vi "Autonomous Independent.vi"() -> ()   [LabVIEW 2018]
doc: "This VI is called when autonomous begins, and will automatically be terminated when autonomous ends. You can carry out timed or sensor driven robot movement independently without needing to return to the caller."
uses:
  <vilib>/Rock Robotics/WPI/Solenoid/WPI_SolenoidValue.ctl
  <vilib>/Rock Robotics/WPI/Utilities/WPI_GetSetVariantRefNum.vi
  <vilib>/Rock Robotics/WPI/Solenoid/WPI_SolenoidSetEnum.vi
  <vilib>/Rock Robotics/Network Tables/NT Write Number.vi
  <vilib>/Rock Robotics/Network Tables/NT Write Boolean Array.vi
  <vilib>/Rock Robotics/Network Tables/NT Write Numeric Array.vi
  <vilib>/Rock Robotics/WPI/RobotDrive/WPI_RobotDriveArcadeDrive_Standard(NoSaturation).vi
  <vilib>/Rock Robotics/Network Tables/NT Read String.vi
panel:
  out "Current Movement, for debugging":T1 {"Y Joystick Value" scale=1.0..-1.0; "X Joystick Value" scale=-1.0..1.0}
  in  "Array of robot movements by from the robot":T2(array[cluster])=[{"X Joystick Value"=0.39393939393939403, "Y Joystick Value"=0.0, "Delay (sec)"=1.0, "Movement Name"="turn"}, {"X Joystick Value"=-0.3737373737373737, "Y Joystick Value"=0.0, "Delay (sec)"=1.0, "Movement Name"="turn back"}] {"Y Joystick Value" scale=1.0..-1.0; "X Joystick Value" scale=-1.0..1.0}
  # "Be sure to right-click and choose Data Operations>>Make Current Value default if you want to save the array values with the VI"
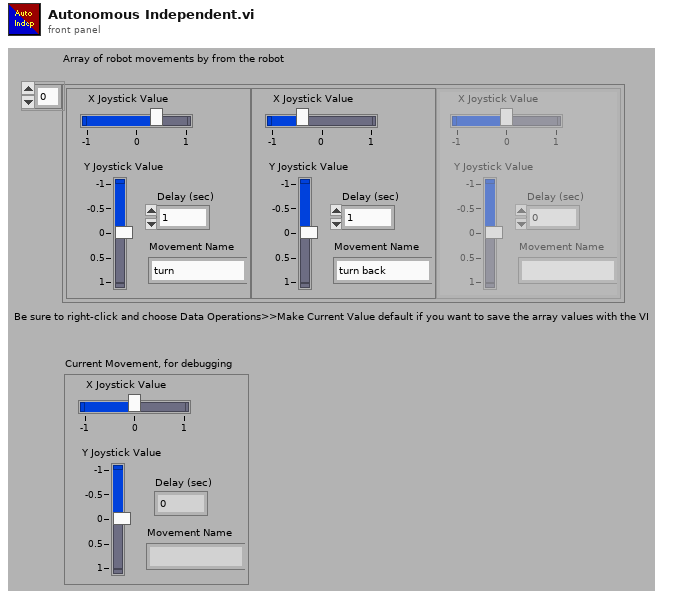
[diagram p1: front panel]
types:
  T1 = cluster{"X Joystick Value":dbl, "Y Joystick Value":dbl, "Delay (sec)":dbl, "Movement Name":string}
  T2 = cluster{"X Joystick Value":dbl, "Y Joystick Value":dbl, "Delay (sec)":dbl, "Movement Name":string}[]
  T3 = typedef "WPI_SolenoidValue.ctl" = enum16{"Off", "On", "Forward", "Reverse"}
  T4 = typedef "WPI_JoystickDevRef.ctl" = cluster{"Device":T5}
  T5 = typedef "WPI_JoystickDeviceEnum.ctl" = enum16{"USB 0", "USB 1", "USB 2", "USB 3", "USB 4", "USB 5"}
  T6 = typedef "WPI_SolenoidDevRef.ctl" = cluster{"DevStatus":errorcluster, "Pneumatics Control Module":u8, "Forward Solenoid Channel":T7, "Reverse Solenoid Channel":T7}
  T7 = typedef "WPI_SolenoidChannel.ctl" = enum8{"Solenoid 0", "Solenoid 1", "Solenoid 2", "Solenoid 3", "Solenoid 4", "Solenoid 5", "Solenoid 6", "Solenoid 7", "Invalid"}
  T8 = typedef "WPI_RobotDriveDevRef.ctl" = cluster{"DevStatus":errorcluster, "Motors[]":T9[], "Square Inputs":bool, "Max Output":dbl}
  T9 = typedef "WPI_MotorControlDeviceRef.ctl" = cluster{"DeviceStatus":errorcluster, "Type":T10, "PWM":cluster{"PWM Channel":T11, "DeadBand":T12}, "CAN":cluster{"Device Number":u8, "SetOutput VI Ref":variant, "GetOutput VI Ref":variant, "Enable VI Ref":variant, "Disable VI Ref":variant, "Data":variant}, "Invert":bool, "DIO PWM":cluster{"PWM \"Enable\" Channel":T11, "DIOChannel":T13, "PWM Rate":dbl}}
  T10 = typedef "WPI_MotorControlType.ctl" = enum16{"PWM", "CAN", "DIO PWM"}
  T11 = typedef "FPGA_DIOPWMChannel.ctl" = enum8{"PWM 0", "PWM 1", "PWM 2", "PWM 3", "PWM 4", "PWM 5", "PWM 6", "PWM 7", "PWM 8", "PWM 9", "PWM MXP 0", "PWM MXP 1", "PWM MXP 2", "PWM MXP 3", "PWM MXP 4", "PWM MXP 5", "PWM MXP 6", "PWM MXP 7", "PWM MXP 8", "PWM MXP 9", "Invalid"}
  T12 = typedef "WPI_PWMDeadband.ctl" = cluster{"Name":string, "maxPositivePwm":i32, "minPositivePwm":i32, "centerPwm":i32, "maxNegativePwm":i32, "minNegativePwm":i32, "angularRange":u16}
  T13 = typedef "FPGA_DIOChannel.ctl" = enum8{"DIO 0", "DIO 1", "DIO 2", "DIO 3", "DIO 4", "DIO 5", "DIO 6", "DIO 7", "DIO 8", "DIO 9", "DIO MXP 0", "DIO MXP 1", "DIO MXP 2", "DIO MXP 3", "DIO MXP 4", "DIO MXP 5", "DIO MXP 6", "DIO MXP 7", "DIO MXP 8", "DIO MXP 9", "DIO MXP 10", "DIO MXP 11", "DIO MXP 12", "DIO MXP 13", "DIO MXP 14", "DIO MXP 15", "SPI Port CS1", "SPI Port CS2", "SPI Port CS3", "SPI Port MISO", "SPI Port MOSI", "Invalid"}
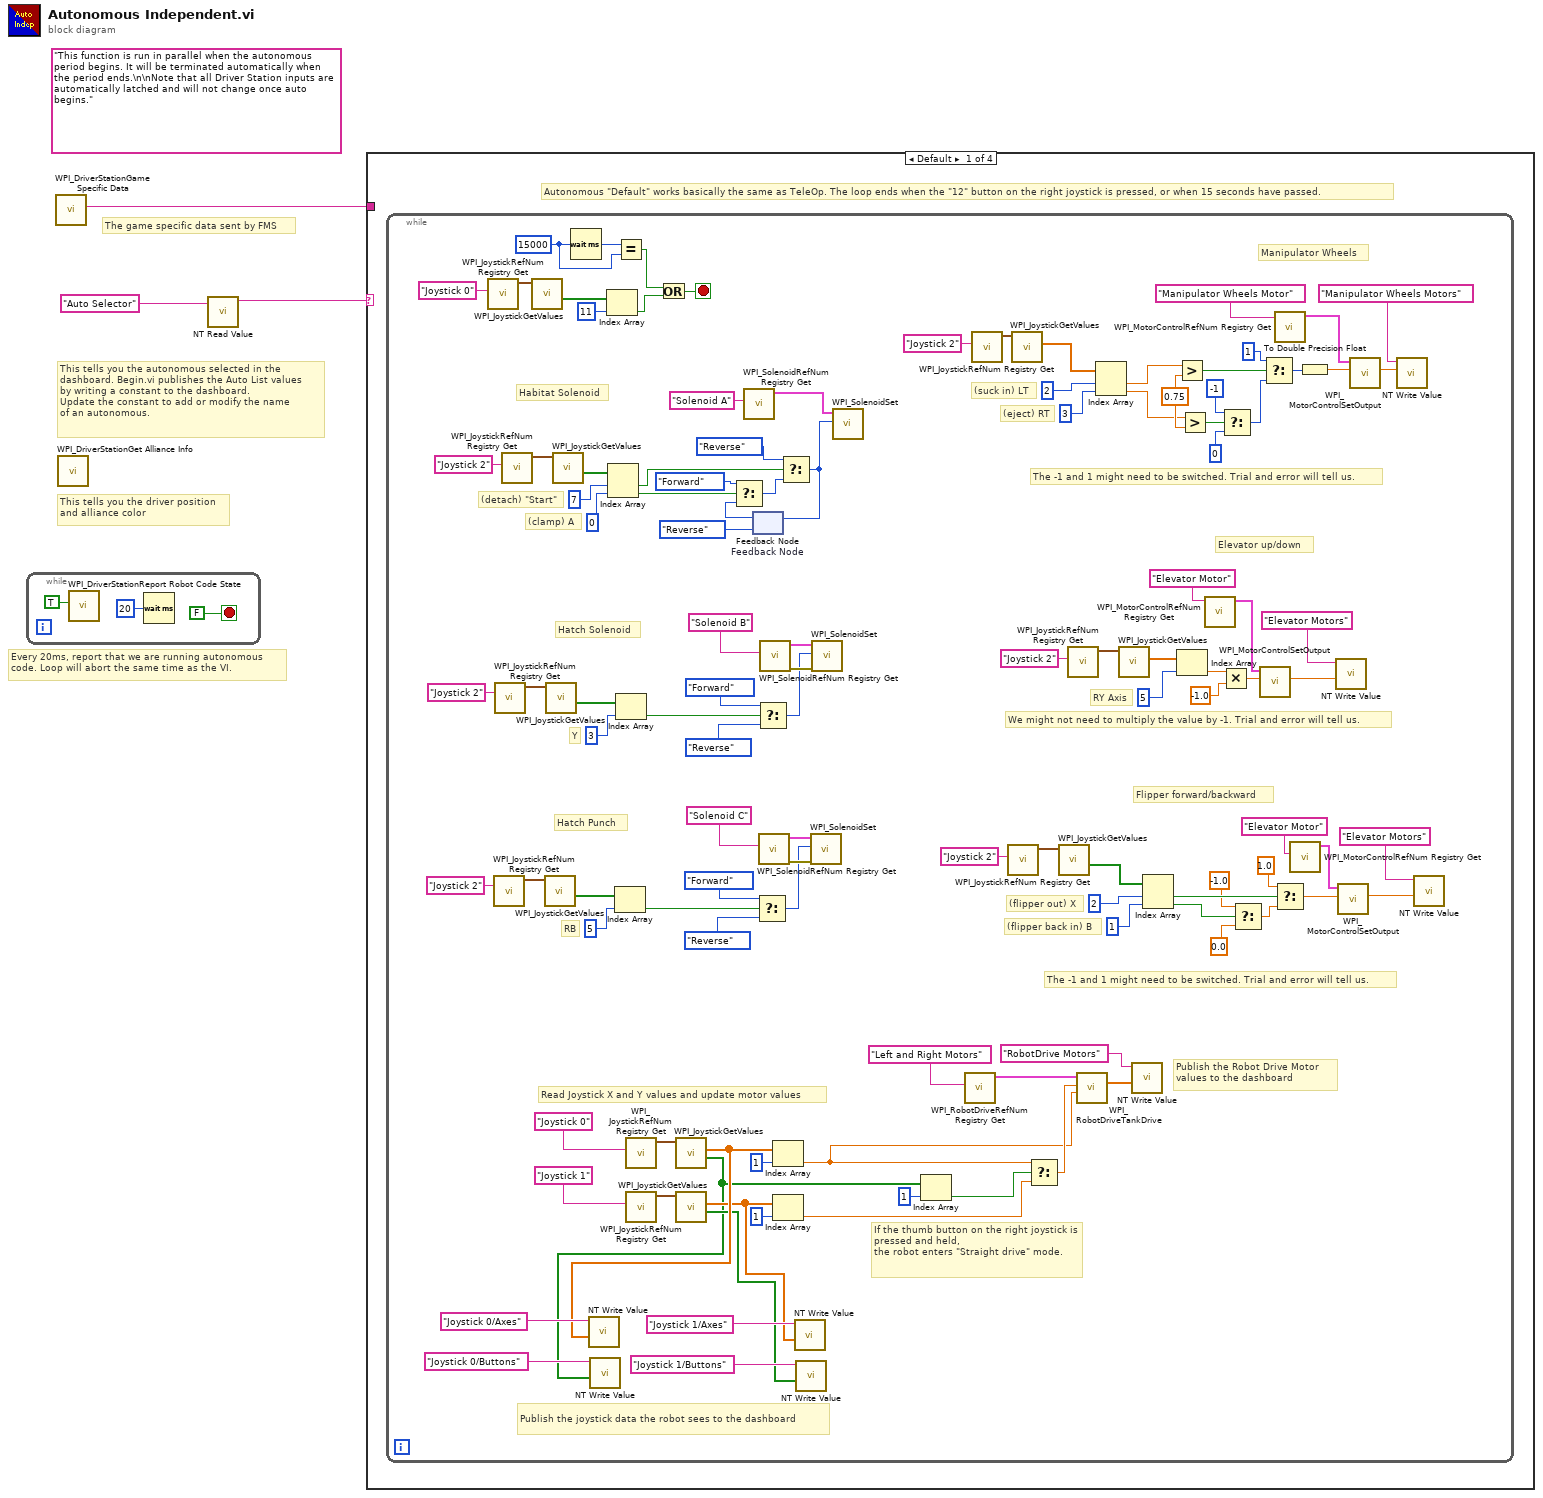
[diagram p0: block diagram]
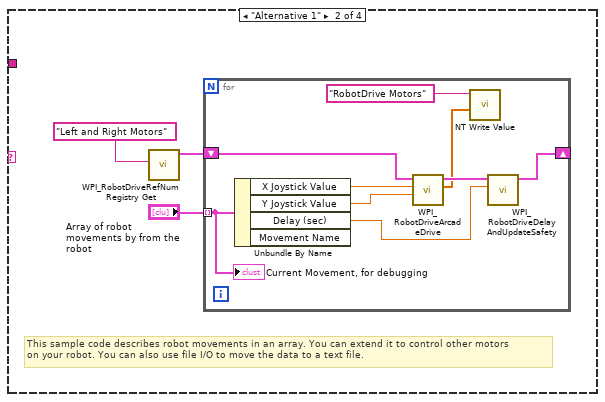
[diagram p2: hidden frame]
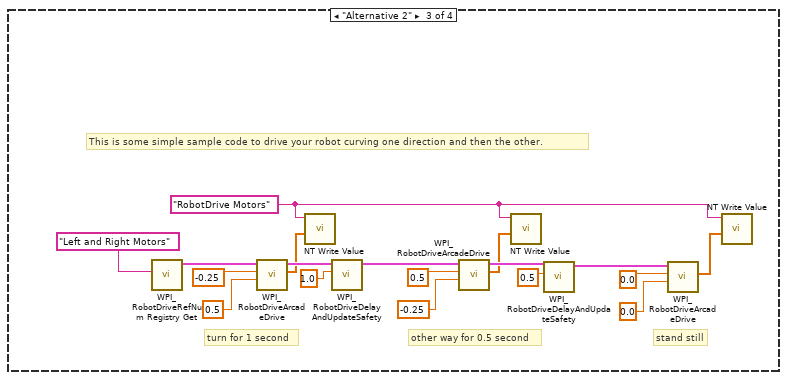
[diagram p3: hidden frame]
diagram:
  (unwired) "This function is run in parallel when the autonomous period begins. It will be terminated automatically when the period ends.\n\nNote that all Driver Station inputs are automatically latched and will not change once auto begins."
  # "The game specific data sent by FMS"
  # "This tells you the autonomous selected in the \ndashboard. Begin.vi publishes the Auto List values\nby writing a constant to the dashboard.\nUpdate the constant to add or modify the name\nof an autonomous."
  # "Every 20ms, report that we are running autonomous\ncode. Loop will abort the same time as the VI."
  # "This tells you the driver position\nand alliance color"
  n1 = while {
    stop <- FALSE stop-if-true
    n2 = call <vilib>:"WPI_DriverStationReport Robot Code State.vi"("Autonomous"=TRUE) -> ()  [unwired: 10 in, 1 out]
    n3 = Wait (ms)(milliseconds to wait=u32 20) -> ()  [unwired: 1 out]
  }
  n4 = call <vilib>:"WPI_DriverStationGame Specific Data.vi"() -> ("Game Specific Data"=w1:string)  [unwired: 11 in]
  n5 = call <vilib>:"WPI_DriverStationGet Alliance Info.vi"() -> ()  [unwired: 12 out]
  n6 = call-poly <vilib>:"NT Read Value.vi"("Name"="Auto Selector") -> ("String"=w2:string)  [unwired: 9 in, 1 out]
  n7 = case shown="Default" w2 {
    tunnel: w1 -> [_ _ _ _]
    frame Default {
      # "Autonomous \"Default\" works basically the same as TeleOp. The loop ends when the \"12\" button on the right joystick is pressed, or when 15 seconds have passed."
      n8 = while {
        stop <- w10 stop-if-true
        w8 = u32 15000 ("milliseconds to wait")
        w75 = 0.75
        # "If the thumb button on the right joystick is pressed and held,\nthe robot enters \"Straight drive\" mode."
        # "Publish the Robot Drive Motor\nvalues to the dashboard"
        # "Publish the joystick data the robot sees to the dashboard"
        # "Read Joystick X and Y values and update motor values"
        # "The -1 and 1 might need to be switched. Trial and error will tell us."
        # "The -1 and 1 might need to be switched. Trial and error will tell us."
        # "Flipper forward/backward"
        # "(flipper back in) B"
        # "(flipper out) X"
        # "We might not need to multiply the value by -1. Trial and error will tell us."
        # "Elevator up/down"
        # "RY Axis"
        # "Manipulator Wheels"
        # "(eject) RT"
        # "(suck in) LT"
        # "RB"
        # "Hatch Punch"
        # "(clamp) A"
        # "(detach) \"Start\""
        # "Y"
        # "Habitat Solenoid"
        # "Hatch Solenoid"
        n9 = call <vilib>:"WPI_JoystickRefNum Registry Get.vi"("refnum name"="Joystick 0") -> ("JoystickDevRef"=w121:T4)  [unwired: 1 in, 9 out]
        n10 = call <vilib>:"WPI_JoystickRefNum Registry Get.vi"("refnum name"="Joystick 2") -> ("JoystickDevRef"=w87:T4)  [unwired: 9 in, 1 out]
        n11 = call <vilib>:"WPI_JoystickRefNum Registry Get.vi"("refnum name"="Joystick 2") -> ("JoystickDevRef"=w113:T4)  [unwired: 9 in, 1 out]
        n12 = call <vilib>:"WPI_JoystickRefNum Registry Get.vi"("refnum name"="Joystick 2") -> ("JoystickDevRef"=w98:T4)  [unwired: 9 in, 1 out]
        n13 = call <vilib>:"WPI_JoystickGetValues.vi"("JoystickDevRef"=w121) -> ("Buttons"=w120:bool[])  [unwired: 6 in, 4 out]
        n14 = call <vilib>:"WPI_JoystickGetValues.vi"("JoystickDevRef"=w87) -> ("Buttons"=w88:bool[])  [unwired: 6 in, 4 out]
        n15 = call <vilib>:"WPI_JoystickGetValues.vi"("JoystickDevRef"=w113) -> ("Buttons"=w114:bool[])  [unwired: 6 in, 4 out]
        n16 = call <vilib>:"WPI_JoystickGetValues.vi"("JoystickDevRef"=w98) -> ("Buttons"=w97:bool[])  [unwired: 6 in, 4 out]
        n17 = Wait (ms)(milliseconds to wait=w8) -> (millisecond timer value=w9:u32)
        n18 = Index Array(array=w120, index=11) -> (element=w11:bool)
        n19 = Index Array "Index Array"(array=w97, index #1=7 ("index"), index #2=0 ("index")) -> (element #1=w94:bool, element #2=w95:bool)
        n20 = Index Array "Index Array"(array=w88, index=5) -> (element=w84:bool)
        n21 = Equal?(x=w9, y=w8) -> (x = y?=w7:bool)
        n22 = Index Array "Index Array"(array=w114, index=3) -> (element=w110:bool)
        n23 = call <vilib>:"WPI_JoystickRefNum Registry Get.vi"("refnum name"="Joystick 0") -> ("JoystickDevRef"=w33:T4)  [unwired: 1 in, 9 out]
        n24 = call <vilib>:"WPI_JoystickRefNum Registry Get.vi"("refnum name"="Joystick 1") -> ("JoystickDevRef"=w24:T4)  [unwired: 1 in, 9 out]
        n25 = Or(x=w7, y=w11) -> (x .or. y?=w10:bool)
        n26 = call <vilib>:"WPI_JoystickGetValues.vi"("JoystickDevRef"=w33) -> ("Buttons"=w12:bool[], "Axes"=w28:dbl[])  [unwired: 6 in, 3 out]
        n27 = call-poly <vilib>:"NT Write Value.vi"("Numeric Array"=w28, "Name"="Joystick 0/Axes") -> ()  [unwired: 9 in, 1 out]
        n28 = call-poly <vilib>:"NT Write Value.vi"("Boolean Array"=w12, "Name"="Joystick 0/Buttons") -> ()  [unwired: 9 in, 1 out]
        n29 = call <vilib>:"WPI_JoystickGetValues.vi"("JoystickDevRef"=w24) -> ("Buttons"=w20:bool[], "Axes"=w21:dbl[])  [unwired: 6 in, 3 out]
        n30 = call <vilib>:"WPI_SolenoidRefNum Registry Get.vi"("refnum name"="Solenoid A") -> ("SolenoidDevRef"=w103:T6)  [unwired: 9 in, 1 out]
        n31 = feedback #1 "Feedback Node"(WPI_SolenoidValue."Reverse" ("Value")) -> (w108:T3)
        n32 = Select(t=WPI_SolenoidValue."Forward" ("Value"), s=w95, f=w108) -> (s? t:f=w96:T3)
        n33 = Select(t=WPI_SolenoidValue."Forward" ("Value"), s=w84, f=WPI_SolenoidValue."Reverse" ("Value")) -> (s? t:f=w83:T3)
        n34 = Select(t=WPI_SolenoidValue."Forward" ("Value"), s=w110, f=WPI_SolenoidValue."Reverse" ("Value")) -> (s? t:f=w109:T3)
        n35 = call <vilib>:"WPI_SolenoidRefNum Registry Get.vi"("refnum name"="Solenoid C") -> ("error out"=w91:errorcluster, "SolenoidDevRef"=w90:T6)  [unwired: 9 in]
        n36 = call <vilib>:"WPI_SolenoidRefNum Registry Get.vi"("refnum name"="Solenoid B") -> ("error out"=w117:errorcluster, "SolenoidDevRef"=w116:T6)  [unwired: 9 in]
        n37 = Index Array(array=w28, index=1) -> (element=w13:dbl)
        n38 = Index Array(array=w21, index=1) -> (element=w14:dbl)
        n39 = Select(t=WPI_SolenoidValue."Reverse" ("Value"), s=w94, f=w96) -> (s? t:f=w106:T3)
        n40 = feedback-in #1(w106) -> ()
        n41 = call-poly <vilib>:"NT Write Value.vi"("Numeric Array"=w21, "Name"="Joystick 1/Axes") -> ()  [unwired: 9 in, 1 out]
        n42 = call-poly <vilib>:"NT Write Value.vi"("Boolean Array"=w20, "Name"="Joystick 1/Buttons") -> ()  [unwired: 9 in, 1 out]
        n43 = call-poly <vilib>:"WPI_SolenoidSet.vi"("error in (no error)"=w91, "Value"=w83, "SolenoidDevRef"=w90) -> ()  [unwired: 7 in, 2 out]
        n44 = call-poly <vilib>:"WPI_SolenoidSet.vi"("error in (no error)"=w117, "Value"=w109, "SolenoidDevRef"=w116) -> ()  [unwired: 7 in, 2 out]
        n45 = call-poly <vilib>:"WPI_SolenoidSet.vi"("Value"=w106, "SolenoidDevRef"=w103) -> ()  [unwired: 8 in, 2 out]
        n46 = Index Array(array=w12, index=1) -> (element=w16:bool)
        n47 = call <vilib>:"WPI_RobotDriveRefNum Registry Get.vi"("refnum name"="Left and Right Motors") -> ("RobotDriveDevRef"=w18:T8)  [unwired: 1 in, 9 out]
        n48 = call <vilib>:"WPI_JoystickRefNum Registry Get.vi"("refnum name"="Joystick 2") -> ("JoystickDevRef"=w80:T4)  [unwired: 9 in, 1 out]
        n49 = call <vilib>:"WPI_JoystickRefNum Registry Get.vi"("refnum name"="Joystick 2") -> ("JoystickDevRef"=w50:T4)  [unwired: 9 in, 1 out]
        n50 = call <vilib>:"WPI_JoystickGetValues.vi"("JoystickDevRef"=w80) -> ("Axes"=w77:dbl[])  [unwired: 6 in, 4 out]
        n51 = Select(t=w13, s=w16, f=w14) -> (s? t:f=w15:dbl)
        n52 = call <vilib>:"WPI_JoystickGetValues.vi"("JoystickDevRef"=w50) -> ("Buttons"=w47:bool[])  [unwired: 6 in, 4 out]
        n53 = call <vilib>:"WPI_JoystickRefNum Registry Get.vi"("refnum name"="Joystick 2") -> ("JoystickDevRef"=w61:T4)  [unwired: 9 in, 1 out]
        n54 = call <vilib>:"WPI_RobotDriveTankDrive.vi"("Right axis value"=w13, "Left axis value"=w15, "RobotDriveDevRef"=w18) -> ("Motor Values"=w30:dbl[])  [unwired: 6 in, 2 out]
        n55 = Index Array "Index Array"(array=w77, index #1=2 ("index"), index #2=3 ("index")) -> (element #1=w76:dbl, element #2=w74:dbl)
        n56 = call <vilib>:"WPI_JoystickGetValues.vi"("JoystickDevRef"=w61) -> ("Axes"=w60:dbl[])  [unwired: 6 in, 4 out]
        n57 = call-poly <vilib>:"NT Write Value.vi"("Numeric Array"=w30, "Name"="RobotDrive Motors") -> ()  [unwired: 9 in, 1 out]
        n58 = Index Array "Index Array"(array=w47, index #1=2 ("index"), index #2=1 ("index")) -> (element #1=w46:bool, element #2=w44:bool)
        n59 = Greater?(x=w76, y=w75) -> (0:w72:bool)
        n60 = Index Array "Index Array"(array=w60, index=5) -> (element=w58:dbl)
        n61 = Greater?(x=w74, y=w75) -> (0:w68:bool)
        n62 = call <vilib>:"WPI_MotorControlRefNum Registry Get.vi"("refnum name"="Elevator Motor") -> ("MotorControlDevRef"=w53:T9)  [unwired: 9 in, 1 out]
        n63 = Multiply(x=w58, y=-1.0) -> (x*y=w52:dbl)
        n64 = Select(t=-1, s=w68, f=0) -> (s? t:f=w35:i32)
        n65 = Select(t=-1.0, s=w44, f=0.0) -> (s? t:f=w42:dbl)
        n66 = call <vilib>:"WPI_MotorControlSetOutput.vi"("Output"=w52, "MotorControlDevRef"=w53) -> ("Motor Output"=w55:dbl)  [unwired: 7 in, 2 out]
        n67 = Select(t=1, s=w72, f=w35) -> (s? t:f=w67:i32)
        n68 = call <vilib>:"WPI_MotorControlRefNum Registry Get.vi"("refnum name"="Manipulator Wheels Motor") -> ("MotorControlDevRef"=w63:T9)  [unwired: 9 in, 1 out]
        n69 = Select(t=1.0, s=w46, f=w42) -> (s? t:f=w38:dbl)
        n70 = call <vilib>:"WPI_MotorControlRefNum Registry Get.vi"("refnum name"="Elevator Motor") -> ("MotorControlDevRef"=w36:T9)  [unwired: 9 in, 1 out]
        n71 = To Double Precision Float(number=w67) -> (double precision float=w66:dbl)
        n72 = call-poly <vilib>:"NT Write Value.vi"("Numeric"=w55, "Name"="Elevator Motors") -> ()  [unwired: 9 in, 1 out]
        n73 = call <vilib>:"WPI_MotorControlSetOutput.vi"("Output"=w38, "MotorControlDevRef"=w36) -> ("Motor Output"=w40:dbl)  [unwired: 7 in, 2 out]
        n74 = call <vilib>:"WPI_MotorControlSetOutput.vi"("Output"=w66, "MotorControlDevRef"=w63) -> ("Motor Output"=w65:dbl)  [unwired: 7 in, 2 out]
        n75 = call-poly <vilib>:"NT Write Value.vi"("Numeric"=w65, "Name"="Manipulator Wheels Motors") -> ()  [unwired: 9 in, 1 out]
        n76 = call-poly <vilib>:"NT Write Value.vi"("Numeric"=w40, "Name"="Elevator Motors") -> ()  [unwired: 9 in, 1 out]
      }
    }
    frame "Alternative 1" {
      # "This sample code describes robot movements in an array. You can extend it to control other motors\non your robot. You can also use file I/O to move the data to a text file."
      n77 = call <vilib>:"WPI_RobotDriveRefNum Registry Get.vi"("refnum name"="Left and Right Motors") -> ("RobotDriveDevRef"=w124:T8)  [unwired: 1 in, 9 out]
      n78 = for {
        shift-right: [w132] -> _
        shift-left: w124 -> [w133]
        tunnel: "Array of robot movements by from the robot" -> [w128] mode=indexing
        n79 = Unbundle By Name(w128) -> ("X Joystick Value"=w131:dbl, "Y Joystick Value"=w130:dbl, "Delay (sec)"=w129:dbl)  [unwired: 1 out]
        n80 = call-poly <vilib>:"WPI_RobotDriveArcadeDrive.vi"("Y axis value"=w130, "X axis value"=w131, "RobotDriveDevRef"=w133) -> ("Motor Values"=w126:dbl[], "RobotDriveDevRef"=w134:T8)  [unwired: 1 in, 6 out]
        n81 = call-poly <vilib>:"NT Write Value.vi"("Numeric Array"=w126, "Name"="RobotDrive Motors") -> ()  [unwired: 9 in, 1 out]
        n82 = call <vilib>:"WPI_RobotDriveDelayAndUpdateSafety.vi"("Delay (s)"=w129, "RobotDriveDevRef"=w134) -> ("RobotDriveDevRef 2"=w132:T8)  [unwired: 8 in, 1 out]
        "Current Movement, for debugging" <- w128
      }
    }
    frame "Alternative 2" {
      w136 = "RobotDrive Motors" ("Name")
      # "This is some simple sample code to drive your robot curving one direction and then the other."
      # "stand still"
      # "other way for 0.5 second"
      # "turn for 1 second"
      n83 = call <vilib>:"WPI_RobotDriveRefNum Registry Get.vi"("refnum name"="Left and Right Motors") -> ("RobotDriveDevRef"=w152:T8)  [unwired: 1 in, 9 out]
      n84 = call-poly <vilib>:"WPI_RobotDriveArcadeDrive.vi"("Y axis value"=0.5 ("X axis value"), "X axis value"=-0.25, "RobotDriveDevRef"=w152) -> ("Motor Values"=w135:dbl[], "RobotDriveDevRef"=w145:T8)  [unwired: 1 in, 6 out]
      n85 = call-poly <vilib>:"NT Write Value.vi"("Numeric Array"=w135, "Name"=w136) -> ()  [unwired: 9 in, 1 out]
      n86 = call <vilib>:"WPI_RobotDriveDelayAndUpdateSafety.vi"("Delay (s)"=1.0, "RobotDriveDevRef"=w145) -> ("RobotDriveDevRef 2"=w146:T8)  [unwired: 8 in, 1 out]
      n87 = call-poly <vilib>:"WPI_RobotDriveArcadeDrive.vi"("Y axis value"=-0.25 ("X axis value"), "X axis value"=0.5, "RobotDriveDevRef"=w146) -> ("Motor Values"=w137:dbl[], "RobotDriveDevRef"=w147:T8)  [unwired: 1 in, 6 out]
      n88 = call-poly <vilib>:"NT Write Value.vi"("Numeric Array"=w137, "Name"=w136) -> ()  [unwired: 9 in, 1 out]
      n89 = call <vilib>:"WPI_RobotDriveDelayAndUpdateSafety.vi"("Delay (s)"=0.5, "RobotDriveDevRef"=w147) -> ("RobotDriveDevRef 2"=w148:T8)  [unwired: 8 in, 1 out]
      n90 = call-poly <vilib>:"WPI_RobotDriveArcadeDrive.vi"("Y axis value"=0.0 ("X axis value"), "X axis value"=0.0, "RobotDriveDevRef"=w148) -> ("Motor Values"=w138:dbl[])  [unwired: 1 in, 7 out]
      n91 = call-poly <vilib>:"NT Write Value.vi"("Numeric Array"=w138, "Name"=w136) -> ()  [unwired: 9 in, 1 out]
    }
    frame "Your Turn" {
    }
  }
